vi "加载测试环境.vi"(0 "输入ini文件地址":path=path "F:/Project/GPRS测试/GPRS测试上位机/GPATS.ini", 1 "error in (no error)":errorcluster caption="错误输入（无错误）") -> (2 "加载成功?":bool=TRUE, 3 "测试环境参数":T1={"串口设置"={"COM号"="", "波特率"=9600, "数据比特"=8, "奇偶"=enum."None", "停止位"=10, "流控制"=0}, "网络参数"={"IP地址"="192.168.1.2", "端口号"=502}, "测试选项"={"指令测试"=FALSE, "特殊功能测试"=FALSE, "数据测试"=FALSE, "心跳包测试"=FALSE, "升级测试"=FALSE, "中心切换测试"=FALSE, "生成报告"=FALSE}} {"串口设置"."流控制" items=["无"=0, "XON/XOFF"=1, "RTS/CTS"=2, "DTR/DSR"=4]; "串口设置"."停止位" items=["1.0"=10, "1.5"=15, "2.0"=20]; "串口设置"."波特率" items=["75"=75, "110"=110, "134"=134, "150"=150, "300"=300, "600"=600, "1200"=1200, "1800"=1800, "2400"=2400, "4800"=4800, "7200"=7200, "9600"=9600, "14400"=14400, "19200"=19200, "28800"=28800, "38400"=38400, "56000"=56000, "57600"=57600, "115200"=115200, "128000"=128000, "230400"=230400]}, 4 "error out":errorcluster caption="错误输出")   [LabVIEW 2015]
uses:
  <vilib>/Utility/config.llb/Read Key (String).vi
  <vilib>/Utility/config.llb/Read Key (U32).vi
  <vilib>/Utility/config.llb/Read Key (Boolean).vi
  <vilib>/Utility/config.llb/NI_LVConfig.lvlib
panel:
  in  "COM号":refnum<visa-resource-name>
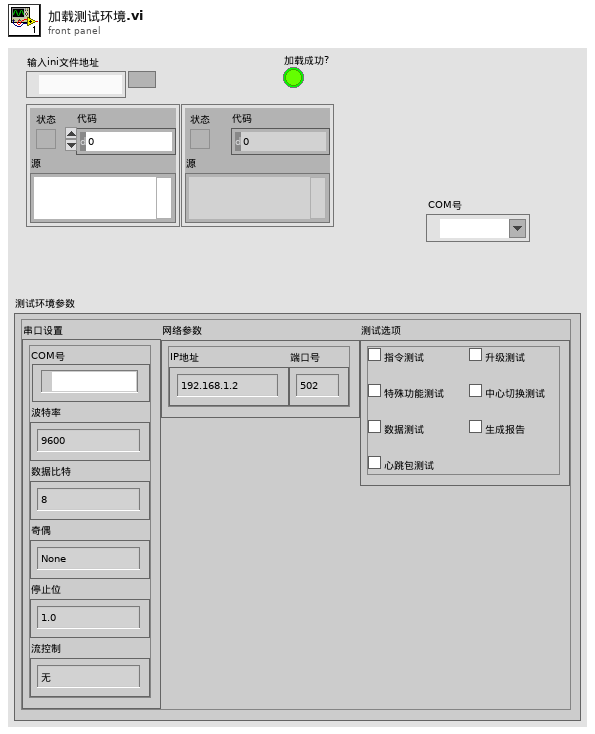
[diagram p1: front panel]
types:
  T1 = typedef "初始化测试环境.ctl" = cluster{"串口设置":T2, "网络参数":T3, "测试选项":T4}
  T2 = typedef "Serial - Settings.ctl" = cluster{"COM号":refnum<visa-resource-name>, "波特率":u32, "数据比特":u16, "奇偶":enum16{"None", "Odd", "Even", "Mark", "Space"}, "停止位":u16, "流控制":u16}
  T3 = typedef "网络参数.ctl" = cluster{"IP地址":string, "端口号":u16}
  T4 = typedef "测试项目.ctl" = cluster{"指令测试":bool, "特殊功能测试":bool, "数据测试":bool, "心跳包测试":bool, "升级测试":bool, "中心切换测试":bool, "生成报告":bool}
  T5 = typedef "NI_LVConfig.lvlib/Config Data RefNum.ctl" = refnum<k1>
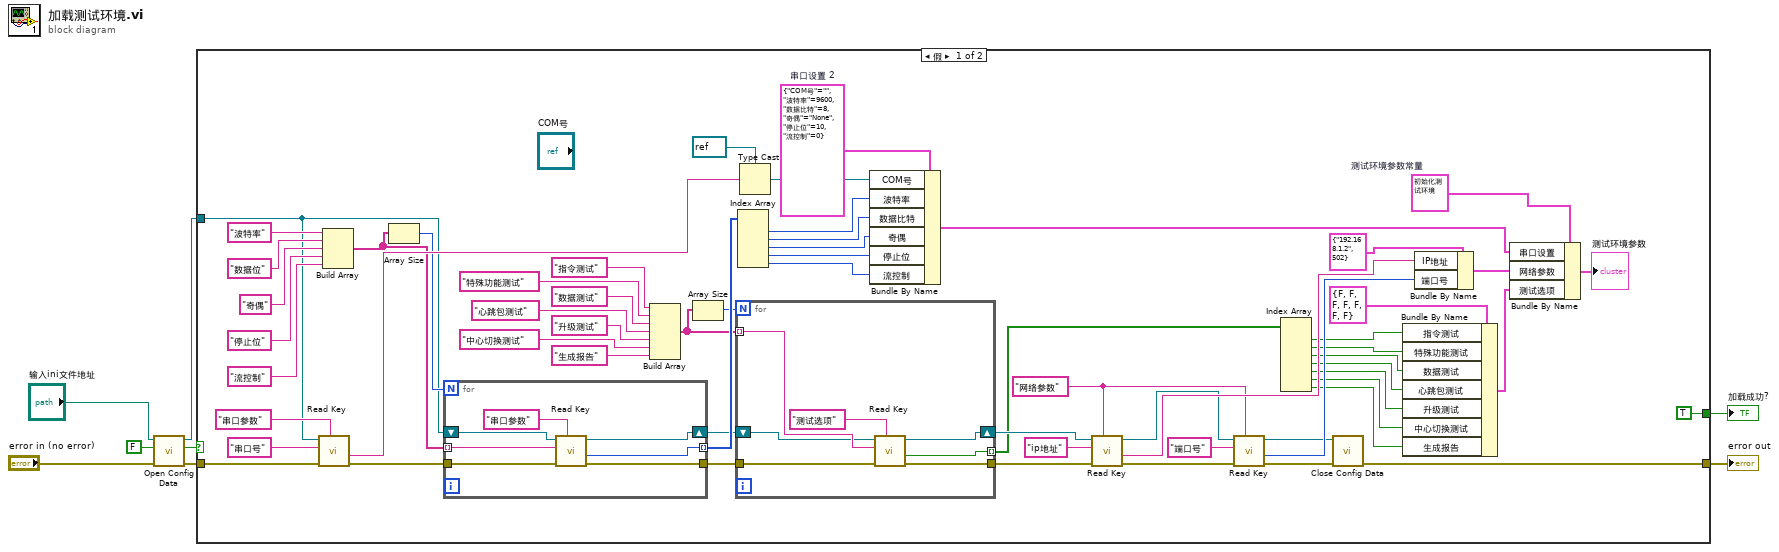
[diagram p0: block diagram]
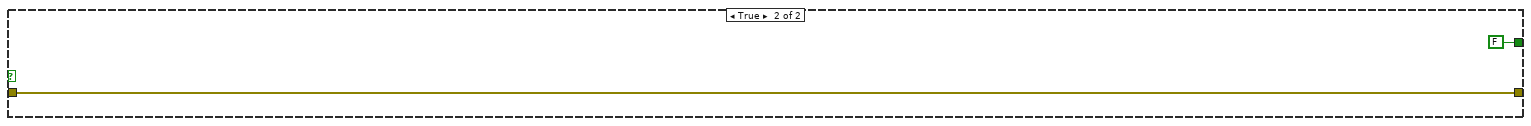
[diagram p2: hidden frame]
diagram:
  n1 = call <vilib>:"Open Config Data.vi"("error in (no error)"="error in (no error)", "create file if necessary (T)"=FALSE, "configuration file path"="输入ini文件地址") -> ("error out"=w8:errorcluster, "file created?"=w4:bool, "refnum"=w5:T5)  [unwired: 6 in]
  n2 = case shown="假" w4 {
    tunnel: w8 -> [w10 w84]
    tunnel: w5 -> [w11 _]
    tunnel: [TRUE FALSE] -> w3
    tunnel: [w68 w84] -> w1
    frame False {
      w9 = T1 {"串口设置"={"COM号"="COM20", "波特率"=1200, "数据比特"=8, "奇偶"=enum."None", "停止位"=10, "流控制"=0}, "网络参数"={"IP地址"="192.168.3.1", "端口号"=5050}, "测试选项"={"指令测试"=TRUE, "特殊功能测试"=TRUE, "数据测试"=TRUE, "心跳包测试"=TRUE, "升级测试"=TRUE, "中心切换测试"=TRUE, "生成报告"=TRUE}}  # 测试环境参数常量
      w16 = "网络参数" ("key")
      w67 = T2 {"COM号"="", "波特率"=9600, "数据比特"=8, "奇偶"=enum."None", "停止位"=10, "流控制"=0}  # 串口设置 2
      n3 = call-poly <vilib>:"Read Key.vi"("section"="串口参数" ("key"), "error in (no error)"=w10, "key"="串口号", "refnum"=w11) -> ("error out"=w37:errorcluster, "value"=w63:string)  [unwired: 4 in, 2 out]
      n4 = Build Array("波特率" ("key"), "数据位" ("key"), "奇偶" ("key"), "停止位" ("key"), "流控制" ("key")) -> (w53:string[])
      n5 = Array Size(array=w53) -> (size(s)=w54:i32)
      n6 = for {
        N: w54 -> [_]
        tunnel: w53 -> [w82] mode=indexing
        tunnel: [w80] -> w52 mode=indexing
        shift-right: [w79] -> w35
        shift-left: w11 -> [w81]
        tunnel: w37 -> [w78]
        tunnel: [w77] -> w36
        n7 = call-poly <vilib>:"Read Key.vi"("section"="串口参数" ("key"), "error in (no error)"=w78, "key"=w82, "refnum"=w81) -> ("error out"=w77:errorcluster, "value"=w80:u32, "refnum out"=w79:T5)  [unwired: 4 in, 1 out]
      }
      n8 = Build Array("指令测试" ("key"), "特殊功能测试" ("key"), "数据测试" ("key"), "心跳包测试" ("key"), "升级测试" ("key"), "中心切换测试" ("key"), "生成报告" ("key")) -> (w40:string[])
      n9 = Array Size(array=w40) -> (size(s)=w41:i32)
      n10 = for {
        N: w41 -> [_]
        tunnel: w40 -> [w76] mode=indexing
        tunnel: [w75] -> w25 mode=indexing
        shift-right: [w74] -> w26
        shift-left: w35 -> [w73]
        tunnel: w36 -> [w72]
        tunnel: [w71] -> w27
        n11 = call-poly <vilib>:"Read Key.vi"("section"="测试选项" ("key"), "error in (no error)"=w72, "key"=w76, "refnum"=w73) -> ("error out"=w71:errorcluster, "value"=w75:bool, "refnum out"=w74:T5)  [unwired: 4 in, 1 out]
      }
      n12 = Index Array(array=w52) -> (element #1=w51:u32, element #2=w50:u32, element #3=w49:u32, element #4=w48:u32, element #5=w47:u32)  [unwired: 5 in]
      n13 = Type Cast(type=refnum<visa-resource-name> refnum ("COM号"), x=w63) -> (*(type *) &x=w61:refnum<visa-resource-name>)
      n14 = Bundle By Name(cluster=w67, "COM号"=w61, "波特率"=w51, "数据比特"=w50, "奇偶"=w49, "停止位"=w48, "流控制"=w47) -> (w14:T2)
      n15 = call-poly <vilib>:"Read Key.vi"("section"=w16, "error in (no error)"=w27, "key"="ip地址", "refnum"=w26) -> ("error out"=w32:errorcluster, "value"=w31:string, "refnum out"=w17:T5)  [unwired: 4 in, 1 out]
      n16 = call-poly <vilib>:"Read Key.vi"("section"=w16, "error in (no error)"=w32, "key"="端口号", "refnum"=w17) -> ("error out"=w29:errorcluster, "value"=w30:u32, "refnum out"=w28:T5)  [unwired: 4 in, 1 out]
      n17 = Index Array(array=w25) -> (element #1=w24:bool, element #2=w23:bool, element #3=w22:bool, element #4=w21:bool, element #5=w20:bool, element #6=w19:bool, element #7=w18:bool)  [unwired: 7 in]
      n18 = call <vilib>:"Close Config Data.vi"("error in (no error)"=w29, "refnum"=w28) -> ("error out"=w68:errorcluster)  [unwired: 8 in, 1 out]
      n19 = Bundle By Name(cluster=T4 {"指令测试"=FALSE, "特殊功能测试"=FALSE, "数据测试"=FALSE, "心跳包测试"=FALSE, "升级测试"=FALSE, "中心切换测试"=FALSE, "生成报告"=FALSE} ("测试选项 2"), "指令测试"=w24, "特殊功能测试"=w23, "数据测试"=w22, "心跳包测试"=w21, "升级测试"=w20, "中心切换测试"=w19, "生成报告"=w18) -> (w12:T4)
      n20 = Bundle By Name(cluster=T3 {"IP地址"="192.168.1.2", "端口号"=502} ("网络信息 2"), "IP地址"=w31, "端口号"=w30) -> (w13:T3)
      n21 = Bundle By Name(cluster=w9, "串口设置"=w14, "网络参数"=w13, "测试选项"=w12) -> (→"测试环境参数":T1)
    }
    frame True {
    }
  }
  "加载成功?" <- w3
  "error out" <- w1
